vi "Read WeatherSensor.lvclass.vi"(8 "error in (no error)":errorcluster, 11 "WeatherStation in":refnum<class "WeatherStation.lvclass">) -> (0 "error out":errorcluster, 2 "WeatherSensor.lvclass":refnum<class "WeatherSensor.lvclass">, 3 "WeatherStation out":refnum<class "WeatherStation.lvclass">)   [LabVIEW 2018, in "WeatherStation.lvclass"]
uses:
  WeatherStation.lvclass
  WeatherSensor/WeatherSensor.lvclass
  WeatherStation.lvclass/WeatherStation.ctl
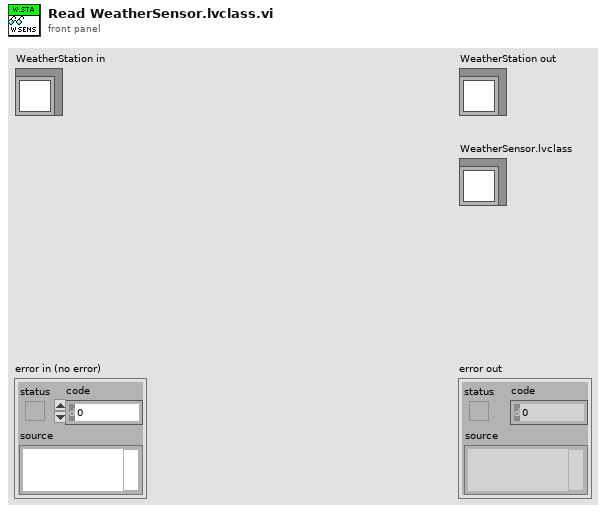
[diagram p1: front panel]
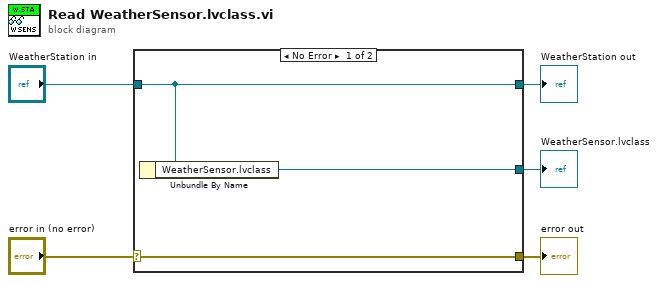
[diagram p0: block diagram]
diagram:
  n1 = case shown="No Error" "error in (no error)" {
    selector: "error in (no error)" -> [w8 w9]
    tunnel: [w8 w9] -> w4
    tunnel: [w7 w10] -> w2
    tunnel: "WeatherStation in" -> [w7 w10]
    tunnel: [w6 _] -> w1
    frame No Error {
      n2 = Unbundle By Name(w7) -> ("WeatherSensor.lvclass"=w6:refnum<class "WeatherSensor.lvclass">)
    }
    frame Error {
    }
  }
  "error out" <- w4
  "WeatherStation out" <- w2
  "WeatherSensor.lvclass" <- w1
